vi "Teste status upload.vi"() -> ()   [LabVIEW 2018, in "Motor.lvclass"]
uses:
  Motor.lvclass
panel:
  in  "download":string[](array[string])
  in  "upload":string[](array[string])
  out "ms upload":u32
  out "error out 2":errorcluster
  out "ms download":u32
  out "error out":errorcluster
  out "ms 5":u32
  out "ms 4":u32
  out "ms 3":u32
  out "PX":string
  out "ms 2":u32
  in  "max value":string="20"
  in  "status in":T1={"mode"="ACTIVE", "condition"="BUSY", "position"="51", "pos_name"="WP2", "pos_id"="2"}
  out "status out":T1
  out "instructions":string[](array[string])
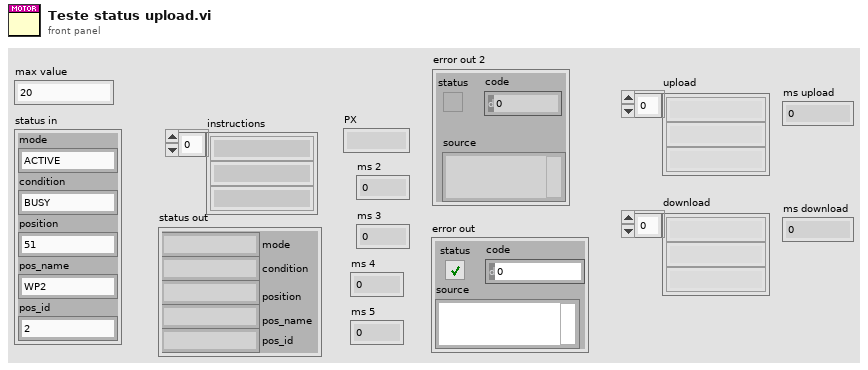
[diagram p1: front panel]
types:
  T1 = cluster{"mode":string, "condition":string, "position":string, "pos_name":string, "pos_id":string}
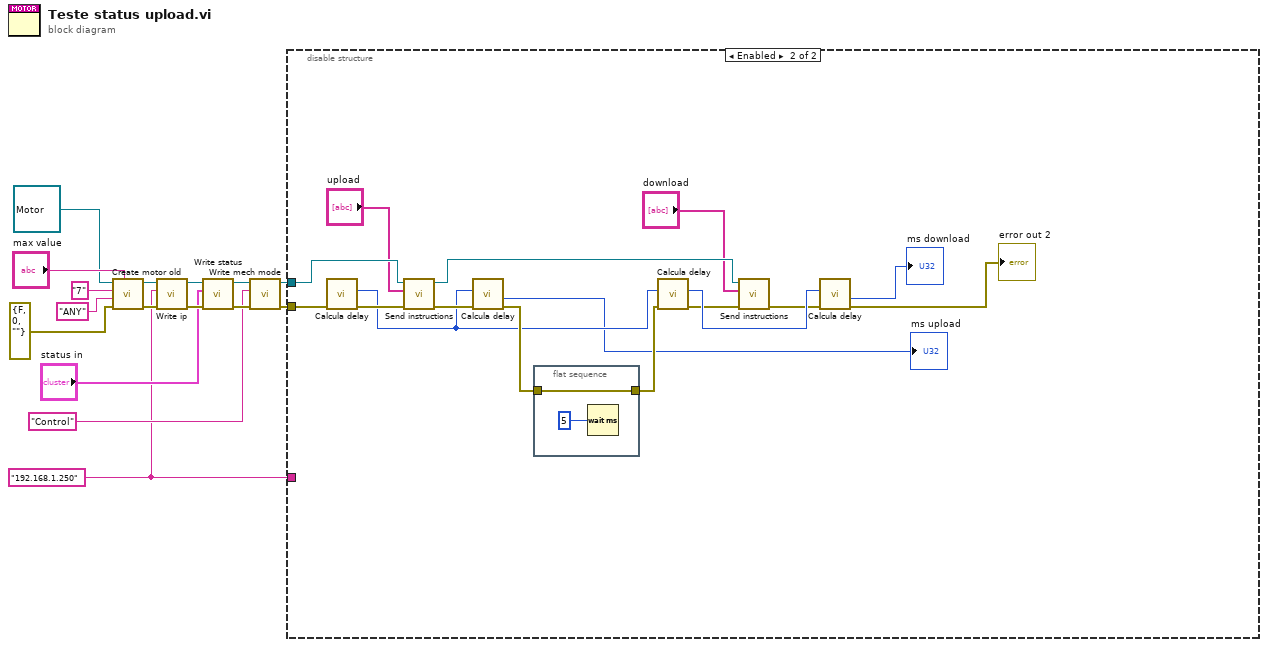
[diagram p0: block diagram]
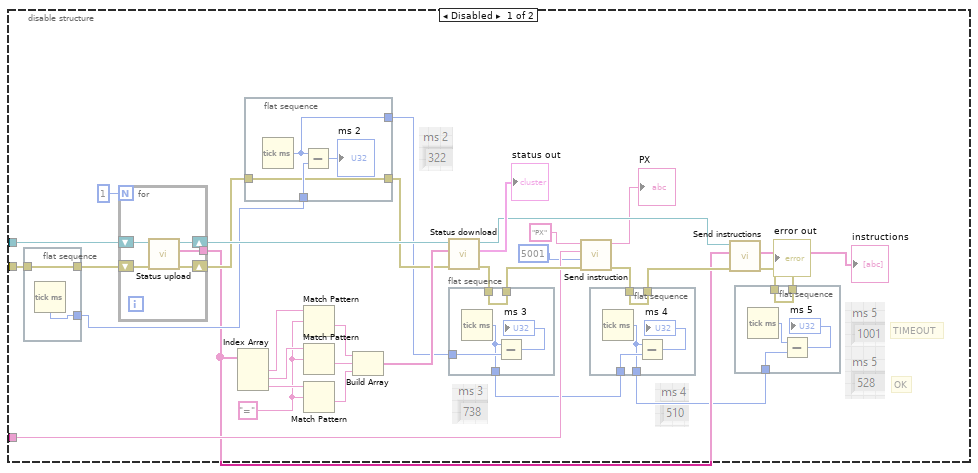
[diagram p2: hidden frame]
diagram:
  w2 = "192.168.1.250" ("ip")
  n1 = call-dynamic "Create motor old.vi"("max param"="max value", "error in (no error)"=errorcluster {"status"=FALSE, "code"=0, "source"=""} ("error out"), "name"="ANY", "id"="7", "Motor in"=refnum<class "Motor.lvclass"> refnum) -> ("error out"=w13:errorcluster, "Motor out"=w12:refnum<class "Motor.lvclass">)  [unwired: 5 in]
  n2 = call-dynamic "Write ip.vi"("error in (no error)"=w13, "ip"=w2, "Motor in"=w12) -> ("error out"=w9:errorcluster, "Motor out"=w10:refnum<class "Motor.lvclass">)  [unwired: 7 in]
  n3 = call-dynamic "Write status.vi"("error in (no error)"=w9, "status"="status in", "Motor in"=w10) -> ("error out"=w5:errorcluster, "Motor out"=w7:refnum<class "Motor.lvclass">)  [unwired: 7 in]
  n4 = call-dynamic "Write mech mode.vi"("error in (no error)"=w5, "mech mode"="Control", "Motor in"=w7) -> ("error out"=w3:errorcluster, "Motor out"=w6:refnum<class "Motor.lvclass">)  [unwired: 7 in]
  n5 = disable-structure shown="Enabled" {
    disable-tunnel: w6 -> [w49 w81]
    disable-tunnel: w3 -> [w38 w88]
    disable-tunnel: w2 -> [w30 _]
    frame Disabled {
      w45 = "="
      # "OK"
      # "TIMEOUT"
      n6 = flat-sequence {
        tunnel: w38 -> [w72]
        tunnel: [w72] -> w37
        tunnel: [w71] -> w33
        frame #0 {
          n7 = Tick Count (ms)() -> (millisecond timer value=w71:u32)
        }
      }
      n8 = for {
        N: 1 -> [_]
        tunnel: [w69] -> w23
        shift-right: [w68] -> w41
        shift-left: w49 -> [w70]
        shift-right: [w67] -> w35
        shift-left: w37 -> [w66]
        n9 = call-dynamic "Status upload.vi"("error in (no error)"=w66, "Motor in"=w70) -> ("error out"=w67:errorcluster, "instructions"=w69:string[], "Motor out"=w68:refnum<class "Motor.lvclass">)  [unwired: 6 in, 1 out]
      }
      n10 = Index Array(array=w23) -> (element #1=w47:string, element #2=w48:string, element #3=w46:string)  [unwired: 3 in]
      n11 = flat-sequence {
        tunnel: w33 -> [w65]
        tunnel: w35 -> [w64]
        tunnel: [w64] -> w34
        tunnel: [w62] -> w27
        frame #0 {
          n12 = Tick Count (ms)() -> (millisecond timer value=w62:u32)
          n13 = Subtract(x=w62, y=w65) -> (x-y=→"ms 2":u32)
        }
      }
      n14 = Match Pattern(string=w47, regular expression=w45) -> (after substring=w42:string)  [unwired: 1 in, 3 out]
      n15 = Match Pattern(string=w48, regular expression=w45) -> (after substring=w44:string)  [unwired: 1 in, 3 out]
      n16 = Match Pattern(string=w46, regular expression=w45) -> (after substring=w43:string)  [unwired: 1 in, 3 out]
      n17 = Build Array(w42, w44, w43) -> (w39:string[])
      n18 = call-dynamic "Status download.vi"("error in (no error)"=w34, "replies"=w39, "Motor in"=w41) -> ("error out"=w32:errorcluster, "status"=→"status out":T1, "Motor out"=w22:refnum<class "Motor.lvclass">)  [unwired: 5 in, 1 out]
      n19 = flat-sequence {
        tunnel: w32 -> [w60]
        tunnel: [w60] -> w31
        tunnel: w27 -> [w59]
        tunnel: [w58] -> w25
        frame #0 {
          n20 = Tick Count (ms)() -> (millisecond timer value=w58:u32)
          n21 = Subtract(x=w58, y=w59) -> (x-y=→"ms 3":u32)
        }
      }
      n22 = call "Send instruction.vi"("error in (no error)"=w31, "motor port"=u16 5001, "motor ip"=w30, "instruction"="PX") -> ("error out"=w26:errorcluster, "response"=→"PX":string)  [unwired: 4 in, 2 out]
      n23 = flat-sequence {
        tunnel: w26 -> [w56]
        tunnel: [w56] -> w24
        tunnel: w25 -> [w55]
        tunnel: [w54] -> w19
        frame #0 {
          n24 = Tick Count (ms)() -> (millisecond timer value=w54:u32)
          n25 = Subtract(x=w54, y=w55) -> (x-y=→"ms 4":u32)
        }
      }
      n26 = call-dynamic "Send instructions.vi"("error in (no error)"=w24, "instructions"=w23, "Motor in"=w22) -> ("error out"=w21:errorcluster, "replies"=→"instructions":string[])  [unwired: 4 in, 3 out]
      n27 = flat-sequence {
        tunnel: w21 -> [w51]
        tunnel: [w51] -> w17
        tunnel: w19 -> [w50]
        frame #0 {
          n28 = Tick Count (ms)() -> (millisecond timer value=w53:u32)
          n29 = Subtract(x=w53, y=w50) -> (x-y=→"ms 5":u32)
        }
      }
      "error out" <- w17
    }
    frame Enabled {
      n30 = call "Calcula delay.vi"("error in"=w88) -> ("error out"=w84:errorcluster, "ms out"=w74:u32)  [unwired: 8 in, 1 out]
      n31 = call-dynamic "Send instructions.vi"("error in (no error)"=w84, "instructions"="upload", "Motor in"=w81) -> ("error out"=w76:errorcluster, "Motor out"=w80:refnum<class "Motor.lvclass">)  [unwired: 4 in, 3 out]
      n32 = call "Calcula delay.vi"("error in"=w76, "ms in"=w74) -> ("error out"=w75:errorcluster, "delay"=→"ms upload":u32)  [unwired: 7 in, 1 out]
      n33 = flat-sequence {
        tunnel: w75 -> [w90]
        tunnel: [w90] -> w77
        frame #0 {
          n34 = Wait (ms)(milliseconds to wait=u32 5) -> ()  [unwired: 1 out]
        }
      }
      n35 = call "Calcula delay.vi"("error in"=w77, "ms in"=w74) -> ("error out"=w83:errorcluster, "ms out"=w87:u32)  [unwired: 7 in, 1 out]
      n36 = call-dynamic "Send instructions.vi"("error in (no error)"=w83, "instructions"="download", "Motor in"=w80) -> ("error out"=w82:errorcluster)  [unwired: 4 in, 4 out]
      n37 = call "Calcula delay.vi"("error in"=w82, "ms in"=w87) -> ("error out"=→"error out 2":errorcluster, "delay"=→"ms download":u32)  [unwired: 7 in, 1 out]
    }
  }
